vi "MotherboardTest - TestStand - Close Termination Monitor.vi"(8 "error in (no error)":errorcluster, 11 "Status Monitor In":T1) -> (0 "error out":errorcluster)   [LabVIEW 2025]
doc: "Closes the execution and termination monitor data property objects the TestStand - Initialize Termination Monitor VI creates."
uses:
  MotherboardTest - TestStand - Status Monitor.ctl
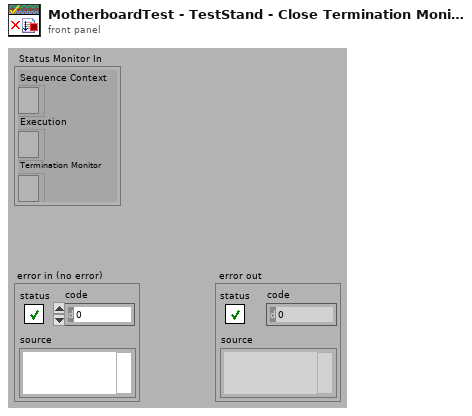
[diagram p1: front panel]
types:
  T1 = typedef "MotherboardTest - TestStand - Status Monitor.ctl" = cluster{"Sequence Context":refnum<k7>, "Execution":refnum<k7>, "Termination Monitor":refnum<k7>}
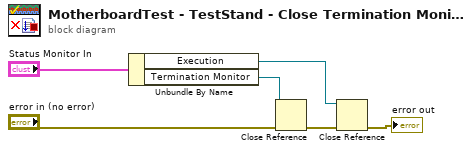
[diagram p0: block diagram]
diagram:
  n1 = Unbundle By Name("Status Monitor In") -> ("Execution"=w4:refnum<k7>, "Termination Monitor"=w5:refnum<k7>)
  n2 = Close Reference(reference=w5, error in (no error)="error in (no error)") -> (error out=w1:errorcluster)
  n3 = Close Reference(reference=w4, error in (no error)=w1) -> (error out=→"error out":errorcluster)
